vi "reg-util-override-duplication.vi"(8 "add timestamp":bool=TRUE, 9 "Rows":i32, 10 "string register":string[](array[string]), 11 "Reports to Collect":string) -> (3 "string register":string[](array[string]))   [LabVIEW 2024]
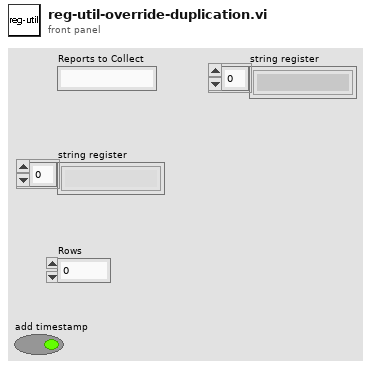
[diagram p1: front panel]
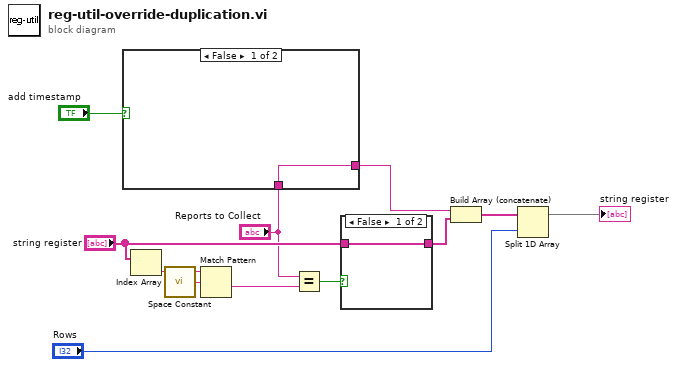
[diagram p0: block diagram]
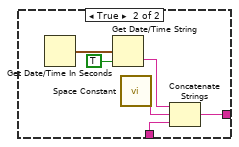
[diagram p2: hidden frame]
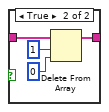
[diagram p3: hidden frame]
diagram:
  n1 = case shown="False" "add timestamp" {
    tunnel: [w13 w16] -> w12
    tunnel: "Reports to Collect" -> [w13 w14]
    frame False {
    }
    frame True {
      n2 = Get Date/Time In Seconds() -> (seconds since 1Jan1904=w19:timestamp)
      n3 = Get Date/Time String(seconds (now)=w19, want seconds? (F)=TRUE) -> (time string=w18:string)  [unwired: 1 in, 1 out]
      n4 = call <vilib>:"Space Constant.vi"() -> ("String"=w15:string)
      n5 = Concatenate Strings(w18, w15, w14) -> (w16:string)
    }
  }
  n6 = Index Array(array="string register") -> (element=w11:string)  [unwired: 1 in]
  n7 = call <vilib>:"Space Constant.vi"() -> ("String"=w10:string)
  n8 = Match Pattern(string=w11, regular expression=w10) -> (after substring=w9:string)  [unwired: 1 in, 3 out]
  n9 = Equal?(x="Reports to Collect", y=w9) -> (x = y?=w8:bool)
  n10 = case shown="False" w8 {
    tunnel: "string register" -> [w20 w24]
    tunnel: [w20 w21] -> w7
    frame False {
    }
    frame True {
      n11 = Delete From Array(array=w24, length=1, index=0) -> (array with subset deleted=w21:string[])  [unwired: 1 out]
    }
  }
  n12 = Build Array (concatenate)(w12, w7) -> (w3:string[])
  n13 = Split 1D Array(array=w3, index="Rows") -> (first subarray=→"string register":string[])  [unwired: 1 out]
